vi "Wavelength iHR320.vi"(8 "error in (no error)":errorcluster, 10 "Spectrometer iHR320.lvclass":refnum<class "Spectrometer iHR320.lvclass">, 11 "Wavelength iHR320.lvclass In":refnum<class "Wavelength iHR320.lvclass">) -> (0 "error out":errorcluster, 3 "Wavelength iHR320.lvclass Out":refnum<class "Wavelength iHR320.lvclass">)   [LabVIEW 2009, in "Wavelength iHR320.lvclass"]
uses:
  Wavelength iHR320.lvclass
  Instruments/Spectrometer iHR320/Spectrometer iHR320.lvclass
  Global/GPIB Numbers.vi
  Wavelength iHR320.lvclass/Wavelength iHR320.ctl
  Scanner/Scanner.lvclass
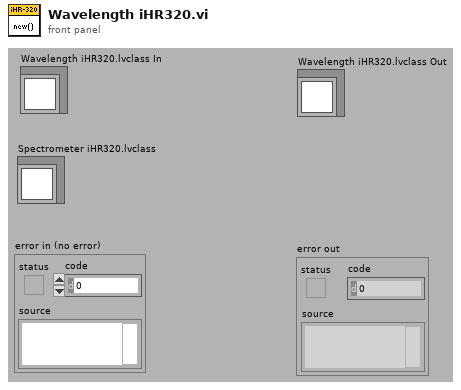
[diagram p1: front panel]
types:
  T1 = typedef "USBMono Type Def.ctl" = cluster{"Name":string, "Unique ID":string}
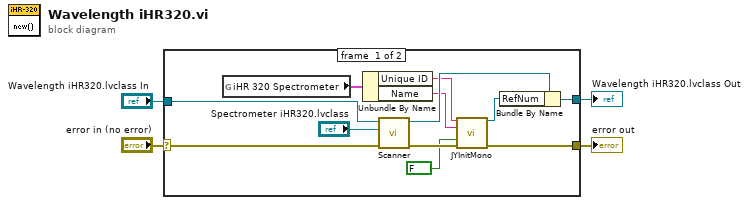
[diagram p0: block diagram]
diagram:
  n1 = case shown="No Error" "error in (no error)" {
    selector: "error in (no error)" -> [w14 w17]
    tunnel: [w9 w17] -> w3
    tunnel: "Wavelength iHR320.lvclass In" -> [w16 w18]
    tunnel: [w11 w18] -> w1
    frame #0 {
      n2 = global read "GPIB Numbers.vi" "iHR 320 Spectrometer"() -> (w12:T1)
      n3 = Unbundle By Name(w12) -> ("Unique ID"=w7:string, "Name"=w6:string)
      n4 = call "Scanner.vi"("error in (no error)"=w14, "Scannable"="Spectrometer iHR320.lvclass", "Scanner.lvclass in"=w16) -> ("error out"=w10:errorcluster, "Scanner.lvclass out"=w13:refnum<class "Wavelength iHR320.lvclass">)  [unwired: 7 in]
      n5 = call "JYInitMono.vi"("Unique ID"=w7, "Mono ID"=w6, "Force Init"=FALSE, "error in (no error)"=w10) -> ("Mono RefNum out"=w8:refnum<k7>, "error out"=w9:errorcluster)  [unwired: 7 in, 3 out]
      n6 = Bundle By Name(cluster=w13, "RefNum"=w8) -> (w11:refnum<class "Wavelength iHR320.lvclass">)
    }
    frame #1 {
    }
  }
  "error out" <- w3
  "Wavelength iHR320.lvclass Out" <- w1
